vi "Java+kill.vi"(8 "error in (no error)":errorcluster) -> (0 "error out":errorcluster)   [LabVIEW 2019]
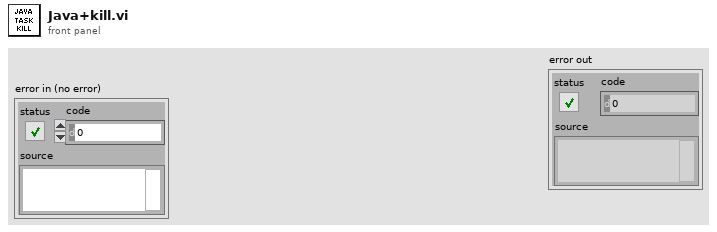
[diagram p1: front panel]
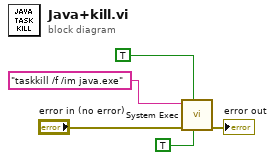
[diagram p0: block diagram]
diagram:
  n1 = call <vilib>:"System Exec.vi"("run minimized? (F)"=TRUE, "wait until completion? (T)"=TRUE, "error in (no error)"="error in (no error)", "command line"="taskkill /f /im java.exe") -> ("error out"=→"error out":errorcluster)  [unwired: 4 in, 3 out]
